vi "Open Model File.vi"(10 "regular expression":string, 11 "All Models Excel Sheet":path) -> (3 "all rows":string[][](array[string]))   [LabVIEW 2012]
doc: "This VI goes to the Model File location and determines if the excel file has been opened before. If it has not been opened before it will pull all of the data out of excel and save the file in the same location in CSV format. This allows for faster processing speeds.\n\nIf it has been opened before, it will open the .csv file"
uses:
  <vilib>/Utility/file.llb/Write To Spreadsheet File (string).vi
  <vilib>/Utility/file.llb/Read From Spreadsheet File (string).vi
panel:
  out "Use Excel":bool
  out "Format 2":string
  out "Format":string
  out "0":bool
  out "1":bool
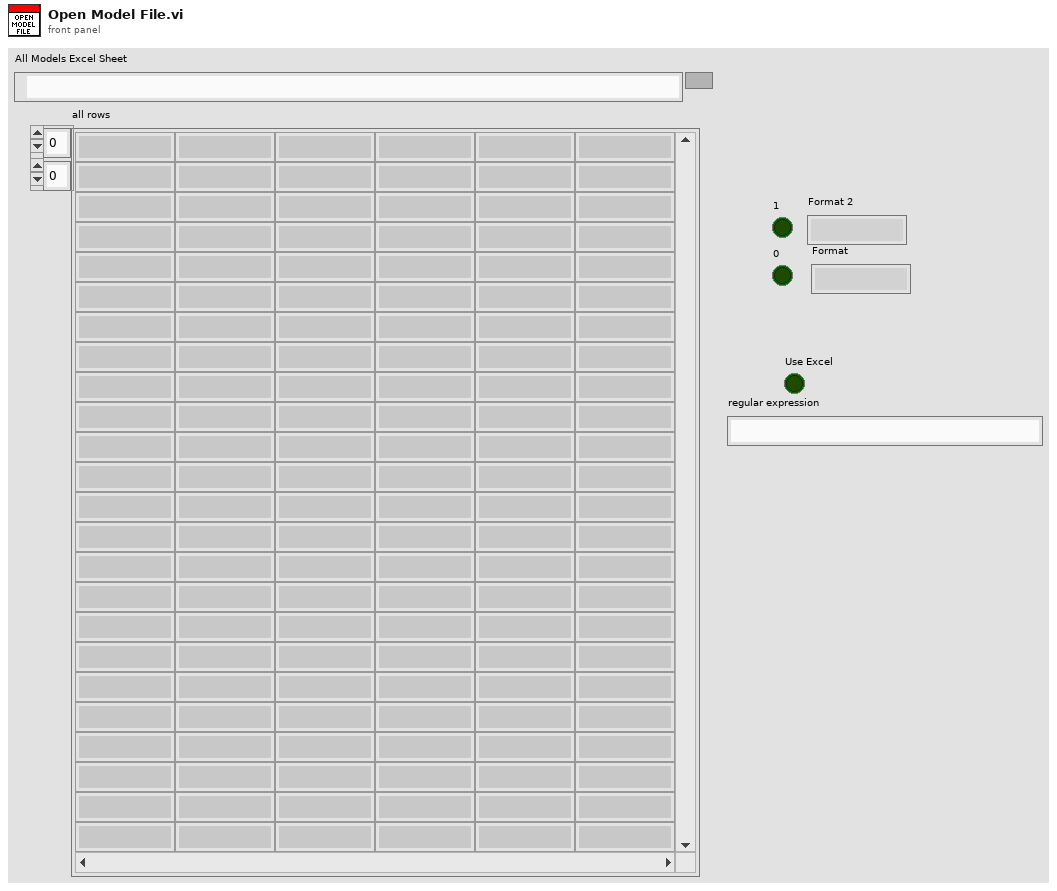
[diagram p1: front panel]
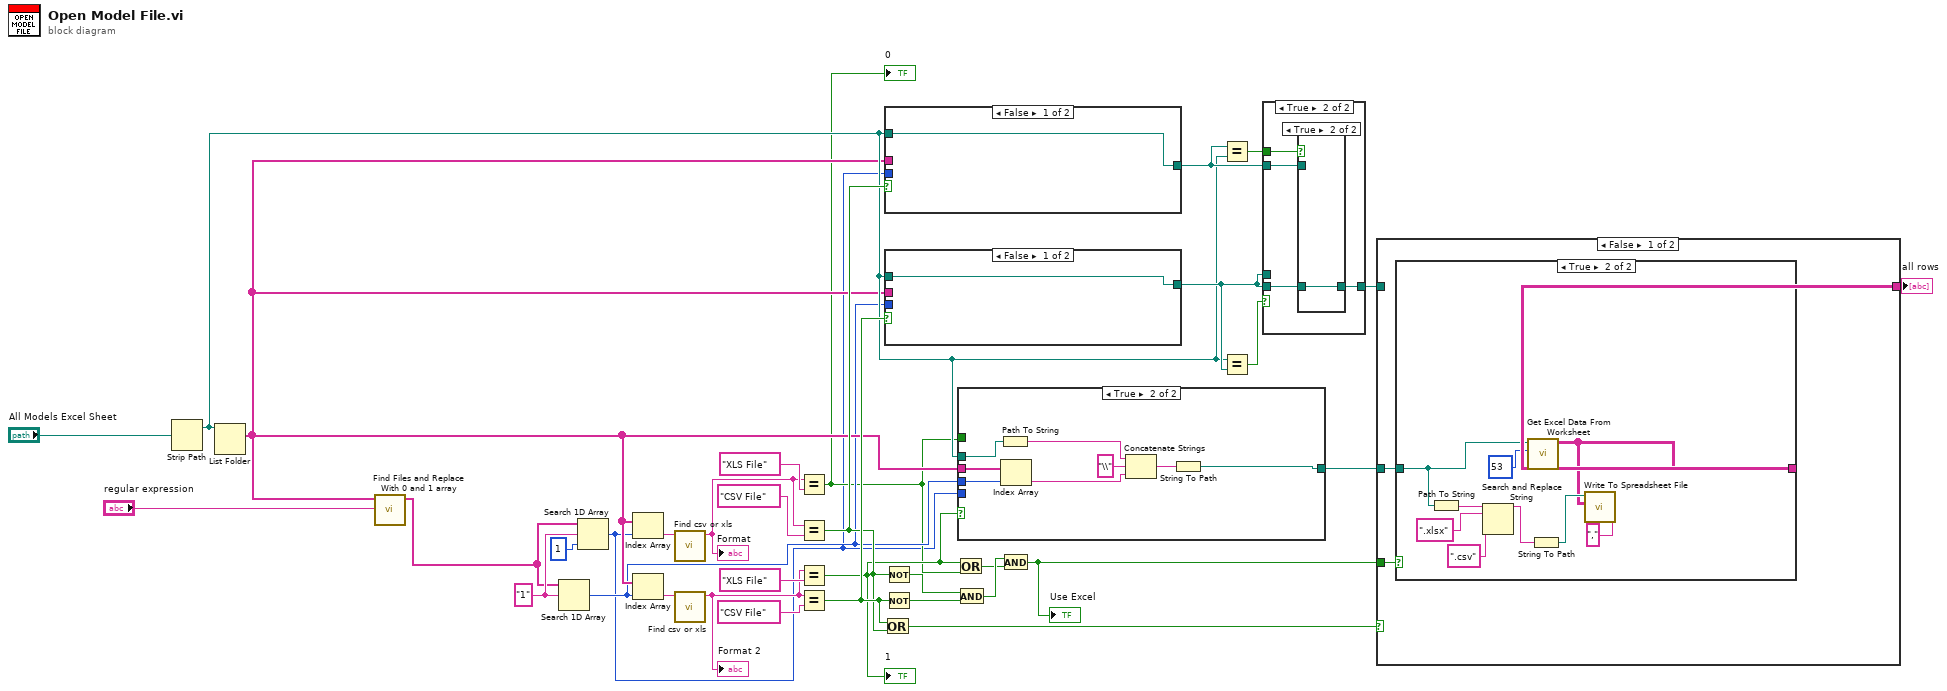
[diagram p0: block diagram]
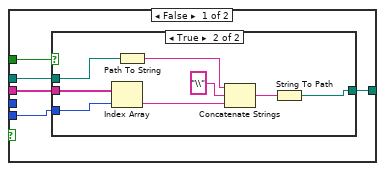
[diagram p2: hidden frame]
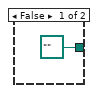
[diagram p3: hidden frame]
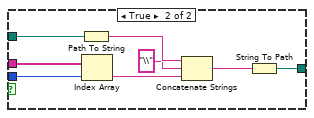
[diagram p6: hidden frame]
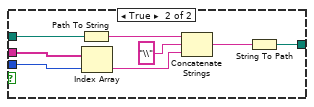
[diagram p7: hidden frame]
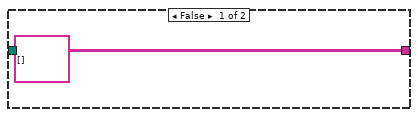
[diagram p8: hidden frame]
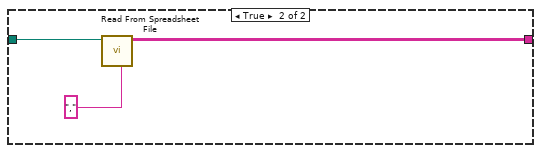
[diagram p9: hidden frame]
diagram:
  w24 = "1" ("element")
  n1 = Strip Path(path="All Models Excel Sheet") -> (stripped path=w7:path)  [unwired: 1 out]
  n2 = List Folder(path=w7) -> (filenames=w6:string[])  [unwired: 3 in, 3 out]
  n3 = call "Find Files and Replace With 0 and 1 array.vi"("regular expression"="regular expression", "filenames"=w6) -> ("Array"=w22:string[])  [unwired: 9 in]
  n4 = Search 1D Array(1D array=w22, element=w24) -> (index of element=w5:i32)  [unwired: 1 in]
  n5 = Search 1D Array(1D array=w22, element=w24, start index (0)=1) -> (index of element=w3:i32)
  n6 = Index Array(array=w6, index=w3) -> (element=w23:string)
  n7 = Index Array(array=w6, index=w5) -> (element=w28:string)
  n8 = call "Find csv or xls.vi"("String"=w23) -> ("Format"=w16:string)  [unwired: 10 in]
  "Format" <- w16
  n9 = call "Find csv or xls.vi"("String"=w28) -> ("Format"=w17:string)  [unwired: 10 in]
  "Format 2" <- w17
  n10 = Equal?(x=w16, y="XLS File") -> (x = y?=w4:bool)
  "0" <- w4
  n11 = Equal?(x=w16, y="CSV File") -> (x = y?=w10:bool)
  n12 = Equal?(x=w17, y="XLS File") -> (x = y?=w8:bool)
  "1" <- w8
  n13 = Equal?(x=w17, y="CSV File") -> (x = y?=w14:bool)
  n14 = Or(x=w14, y=w10) -> (x .or. y?=w27:bool)
  n15 = Not(x=w10) -> (.not. x?=w15:bool)
  n16 = Not(x=w14) -> (.not. x?=w13:bool)
  n17 = case shown="False" w10 {
    tunnel: w6 -> [_ w43]
    tunnel: w3 -> [_ w42]
    tunnel: w7 -> [w35 w41]
    tunnel: [w35 w36] -> w32
    frame False {
    }
    frame True {
      n18 = Path To String(path=w41) -> (string=w40:string)
      n19 = Index Array(array=w43, index=w42) -> (element=w38:string)
      n20 = Concatenate Strings(w40, "\\" ("string"), w38) -> (w37:string)
      n21 = String To Path(string=w37) -> (path=w36:path)
    }
  }
  n22 = case shown="False" w14 {
    tunnel: w6 -> [_ w52]
    tunnel: w5 -> [_ w51]
    tunnel: w7 -> [w44 w50]
    tunnel: [w44 w45] -> w33
    frame False {
    }
    frame True {
      n23 = Path To String(path=w50) -> (string=w49:string)
      n24 = Index Array(array=w52, index=w51) -> (element=w47:string)
      n25 = Concatenate Strings(w49, "\\" ("string"), w47) -> (w46:string)
      n26 = String To Path(string=w46) -> (path=w45:path)
    }
  }
  n27 = Or(x=w8, y=w4) -> (x .or. y?=w11:bool)
  n28 = And(x=w15, y=w13) -> (x .and. y?=w12:bool)
  n29 = case shown="True" w8 {
    tunnel: w7 -> [w55 w70]
    tunnel: w6 -> [w54 w69]
    tunnel: w5 -> [_ w68]
    tunnel: [w57 w67] -> w2
    tunnel: w4 -> [w56 _]
    tunnel: w3 -> [w53 _]
    frame False {
      n30 = case shown="True" w56 {
        tunnel: [path "" w63] -> w57
        tunnel: w55 -> [_ w62]
        tunnel: w54 -> [_ w61]
        tunnel: w53 -> [_ w60]
        frame False {
        }
        frame True {
          n31 = Index Array(array=w61, index=w60) -> (element=w59:string)
          n32 = Path To String(path=w62) -> (string=w64:string)
          n33 = Concatenate Strings(w64, "\\" ("string"), w59) -> (w66:string)
          n34 = String To Path(string=w66) -> (path=w63:path)
        }
      }
    }
    frame True {
      n35 = Path To String(path=w70) -> (string=w71:string)
      n36 = Index Array(array=w69, index=w68) -> (element=w73:string)
      n37 = Concatenate Strings(w71, "\\" ("string"), w73) -> (w74:string)
      n38 = String To Path(string=w74) -> (path=w67:path)
    }
  }
  n39 = And(x=w12, y=w11) -> (x .and. y?=w9:bool)
  "Use Excel" <- w9
  n40 = Equal?(x=w32, y=w7) -> (x = y?=w30:bool)
  n41 = Equal?(x=w7, y=w33) -> (x = y?=w29:bool)
  n42 = case shown="True" w29 {
    tunnel: w30 -> [_ w79]
    tunnel: w33 -> [w75 _]
    tunnel: [w75 w77] -> w31
    tunnel: w32 -> [_ w78]
    tunnel: w33 -> [_ w76]
    frame False {
    }
    frame True {
      n43 = case shown="True" w79 {
        tunnel: w78 -> [w80 _]
        tunnel: [w80 w81] -> w77
        tunnel: w76 -> [_ w81]
        frame False {
        }
        frame True {
        }
      }
    }
  }
  n44 = case shown="False" w27 {
    tunnel: w31 -> [_ w97]
    tunnel: [w82 w96] -> w34
    tunnel: w9 -> [w84 _]
    tunnel: w2 -> [w83 _]
    frame False {
      n45 = case shown="True" w84 {
        tunnel: w83 -> [_ w94]
        tunnel: [string[][] [] ("output array 3") w88] -> w82
        frame False {
        }
        frame True {
          n46 = Path To String(path=w94) -> (string=w93:string)
          n47 = Search and Replace String(input string=w93, search string=".xlsx", replace string=".csv" ("replace string (\"\")")) -> (result string=w90:string)  [unwired: 5 in, 3 out]
          n48 = call "Get Excel Data From Worksheet.vi"("Number of Columns"=53, "template (empty)"=w94) -> ("Array"=w88:string[][])  [unwired: 8 in, 1 out]
          n49 = String To Path(string=w90) -> (path=w89:path)
          n50 = call-poly <vilib>:"Write To Spreadsheet File.vi"("delimiter (\\t)"="," ("delimiter (\\t)"), "2D data"=w88, "file path (dialog if empty)"=w89) -> ()  [unwired: 5 in, 1 out]
        }
      }
    }
    frame True {
      n51 = call-poly <vilib>:"Read From Spreadsheet File.vi"("delimiter (\\t)"="," ("delimiter (\\t)"), "file path (dialog if empty)"=w97) -> ("all rows"=w96:string[][])  [unwired: 5 in, 4 out]
    }
  }
  "all rows" <- w34
